vi "Tx UDP Parameter Conversion.vi"() -> ()   [LabVIEW 2020]
uses:
  d3b482b5-ec9a-491d-b3ca-0ed132300875.vi
  f12c67c0-482f-47fe-bab3-858b04418264.vi
  niveristand-aim-milStd1553-custom-device/Source/Custom Device Support/Shared/Parameter Definition.ctl
panel:
  in  "number of words":u16
  in  "parameters":T1[](array[typedef])
  in  "value index":i32
  out "error out":errorcluster
  in  "error in":errorcluster
  in  "values":dbl[](array[numeric])
  out "data words":u16[](array[numeric]) format="%04x"
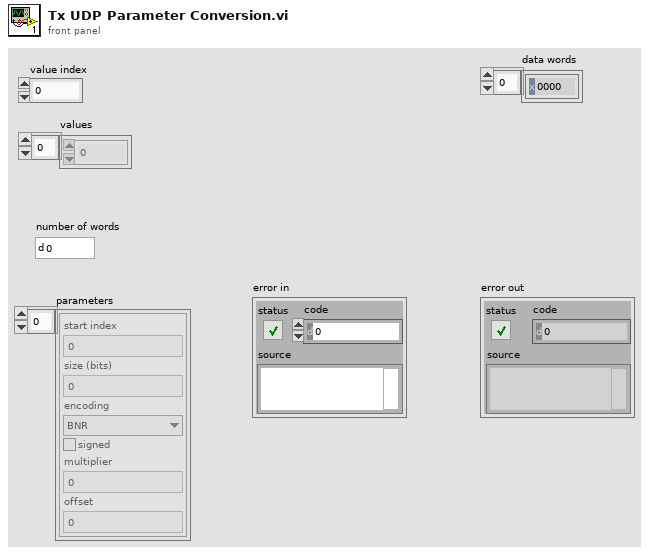
[diagram p1: front panel]
types:
  T1 = typedef "Parameter Definition.ctl" = cluster{"start index":i32, "size (bits)":i32, "encoding":enum16{"BNR", "BCD", "Discrete"}, "signed":bool, "multiplier":dbl, "offset":dbl}
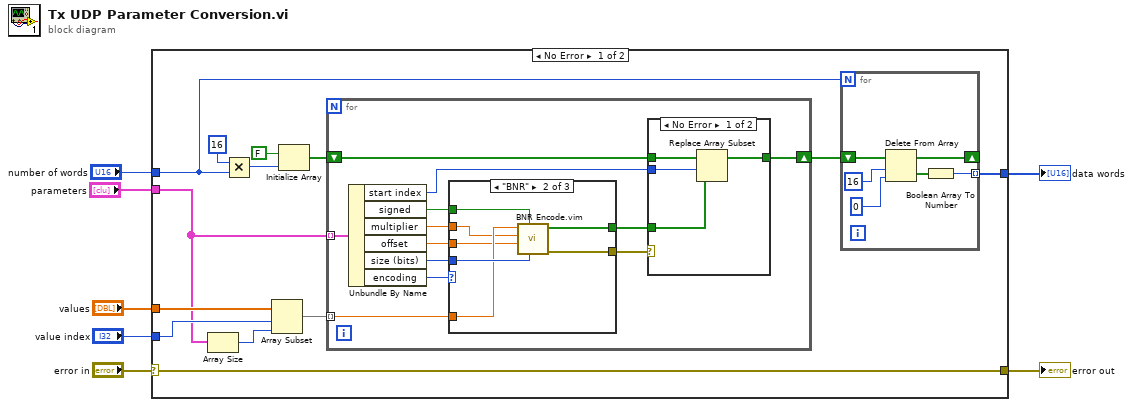
[diagram p0: block diagram]
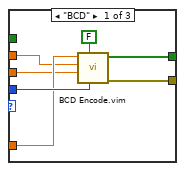
[diagram p3: hidden frame]
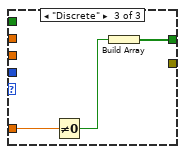
[diagram p4: hidden frame]
diagram:
  n1 = case shown="No Error" "error in" {
    selector: "error in" -> [w11 w61]
    tunnel: "parameters" -> [w9 _]
    tunnel: [w11 w61] -> w6
    tunnel: [w10 _] -> w5
    tunnel: "values" -> [w14 _]
    tunnel: "value index" -> [w13 _]
    tunnel: "number of words" -> [w8 _]
    frame No Error {
      n2 = Array Size(array=w9) -> (size(s)=w12:i32)
      n3 = Multiply(x=u16 16, y=w8) -> (x*y=w19:u16)
      n4 = Array Subset(array=w14, index=w13, length=w12) -> (w15:dbl[])
      n5 = Initialize Array(FALSE, w19) -> (w17:bool[])
      n6 = for {
        shift-right: [w28] -> w16
        shift-left: w17 -> [w29]
        tunnel: w9 -> [w38] mode=indexing
        tunnel: w15 -> [w37] mode=indexing
        n7 = Unbundle By Name(w38) -> ("start index"=w30:i32, "signed"=w35:bool, "multiplier"=w34:dbl, "offset"=w33:dbl, "size (bits)"=w32:i32, "encoding"=w36:enum16{"BNR", "BCD", "Discrete"})
        n8 = case shown="\"BNR\"" w36 {
          tunnel: w37 -> [w48 w54 w60]
          tunnel: w35 -> [_ w57 _]
          tunnel: w34 -> [w47 w53 _]
          tunnel: w33 -> [w46 w52 _]
          tunnel: w32 -> [w49 w55 _]
          tunnel: [w45 w56 _] -> w27
          tunnel: [w44 w51 w59] -> w31
          frame "BCD" {
            n9 = call "BCD Encode.vim"("data size (bits)"=w49, "signed"=FALSE, "scale offset"=w46, "scale multiplier"=w47, "value"=w48) -> ("error out"=w45:errorcluster, "BCD encoded value"=w44:bool[])  [unwired: 4 in, 1 out]
          }
          frame "BNR" {
            n10 = call "BNR Encode.vim"("data size (bits)"=w55, "signed"=w57, "scale offset"=w52, "scale multiplier"=w53, "value"=w54) -> ("error out"=w56:errorcluster, "BNR encoded value"=w51:bool[])  [unwired: 5 in]
          }
          frame "Discrete" {
            n11 = Not Equal To 0?(x=w60) -> (x != 0?=w58:bool)
            n12 = Build Array(w58) -> (w59:bool[])
          }
        }
        n13 = case shown="No Error" w27 {
          tunnel: w31 -> [w42 _]
          tunnel: w30 -> [w41 _]
          tunnel: w29 -> [w40 w43]
          tunnel: [w39 w43] -> w28
          frame No Error {
            n14 = Replace Array Subset(array=w40, new element=w42, index=w41) -> (w39:bool[])
          }
          frame Error {
            # "use previous value on error"
          }
        }
      }
      n15 = for {
        N: w8 -> [_]
        shift-right: [w25] -> _
        shift-left: w16 -> [w26]
        tunnel: [w21] -> w10 mode=indexing
        n16 = Delete From Array(array=w26, length=16 ("index"), index=0) -> (deleted portion=w22:bool[], array with subset deleted=w25:bool[])
        n17 = Boolean Array To Number(Boolean array=w22) -> (number=w21:u16)
      }
    }
    frame Error {
    }
  }
  "data words" <- w5
  "error out" <- w6
